vi "SimulateButtonPress.vi"(8 "Reference to Button":refnum<vi>, 11 "VI Reference":refnum<vi>) -> ()   [LabVIEW 2020, in "MacroAssert.lvlib"]
uses:
  MacroAssert.lvlib
  user32.dll
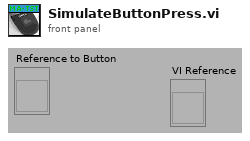
[diagram p1: front panel]
types:
  T1 = typedef "LVRectTypeDef.ctl" = cluster{"Left":i16, "Top":i16, "Right":i16, "Bottom":i16}
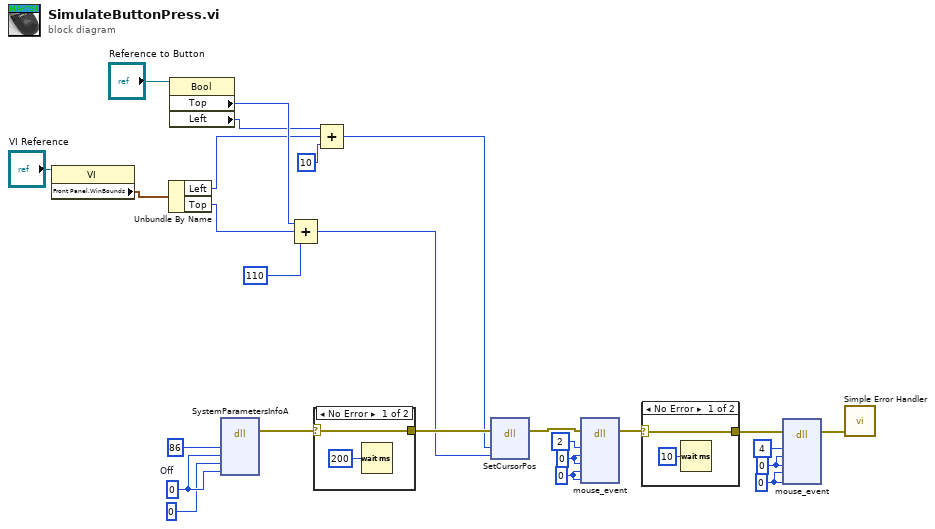
[diagram p0: block diagram]
diagram:
  w24 = 0 ("dwExtraInfo")
  w25 = u32 0 ("dwExtraInfo")
  w23 = 0 ("dwExtraInfo")
  w22 = u32 0 ("dwExtraInfo")
  w20 = u32 0  # Off
  n1 = property class="VI"(reference="VI Reference") -> ("Front Panel.WinBounds"=w11:T1)  [unwired: 1 in, 2 out]
  n2 = Unbundle By Name(w11) -> ("Left"=w3:i16, "Top"=w8:i16)
  n3 = property on="Property Node" class="Bool"(reference="Reference to Button") -> ("Top"=w9:i32, "Left"=w4:i32)  [unwired: 1 in, 2 out]
  n4 = dll-call lib="User32.dll" fn="SystemParametersInfoA" label="Terminate power-off mode"("uiAction"=u32 86 ("SPI_GETPOWEROFFACTIVE"), "uiParam"=w20, "pvParam"=0, "fWinIni"=w20) -> (error out=w17:errorcluster)  [unwired: 8 in, 1 out]
  n5 = Compound Arithmetic op=ADD(w9, w8, 110 ("Position:Left")) -> (w7:i32)
  n6 = case shown="No Error" w17 {
    selector: w17 -> [w27 w29]
    tunnel: [w27 w29] -> w16
    frame No Error {
      n7 = Wait (ms)(milliseconds to wait=u32 200) -> ()  [unwired: 1 out]
    }
    frame Error {
    }
  }
  n8 = Compound Arithmetic op=ADD(w4, w3, i16 10 ("value")) -> (w2:i32)
  n9 = dll-call lib="User32.dll" fn="SetCursorPos" label="Move mouse"(error in=w16, "dx"=w2, "dy"=w7) -> (error out=w15:errorcluster)  [unwired: 5 in, 1 out]
  n10 = dll-call lib="User32.dll" fn="mouse_event" label="Click"(error in=w15, "dwFlags"=2, "dx"=w23, "dy"=w23, "dwData"=w22, "dwExtraInfo"=w22) -> (error out=w14:errorcluster)  [unwired: 8 in, 1 out]
  n11 = case shown="No Error" w14 {
    selector: w14 -> [w30 w32]
    tunnel: [w30 w32] -> w13
    frame No Error {
      n12 = Wait (ms)(milliseconds to wait=u32 10) -> ()  [unwired: 1 out]
    }
    frame Error {
    }
  }
  n13 = dll-call lib="User32.dll" fn="mouse_event" label="Release"(error in=w13, "dwFlags"=4, "dx"=w24, "dy"=w24, "dwData"=w25, "dwExtraInfo"=w25) -> (error out=w12:errorcluster)  [unwired: 8 in, 1 out]
  n14 = call <vilib>:"Simple Error Handler.vi"("error in (no error)"=w12) -> ()  [unwired: 4 in, 5 out]
